vi "Run Sequence.vi"(8 "error in (no error)":errorcluster, 11 "Sequence in":refnum<class "Sequence.lvclass">) -> (0 "error out":errorcluster, 3 "Sequence out":refnum<class "Sequence.lvclass">)   [LabVIEW 2015, in "Mediator.lvlib" / "Sequence.lvclass"]
doc: "This executes the sequence by reserving each step's resources, executing each step, and unreserving each step's resources."
uses:
  Sequence.lvclass
  Sequence.lvclass/Sequence.ctl
  Step/Step.lvclass
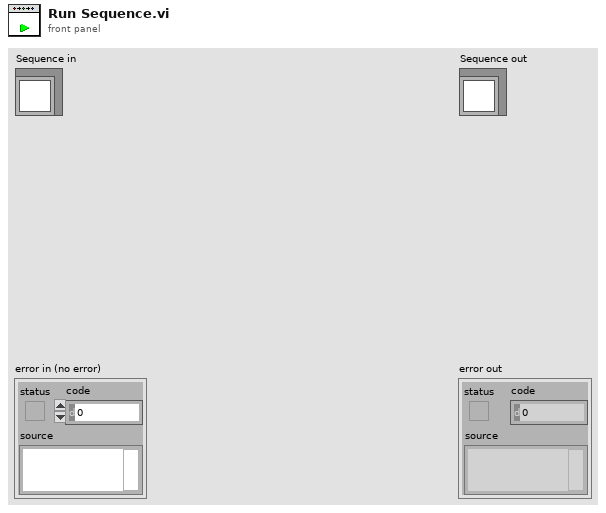
[diagram p1: front panel]
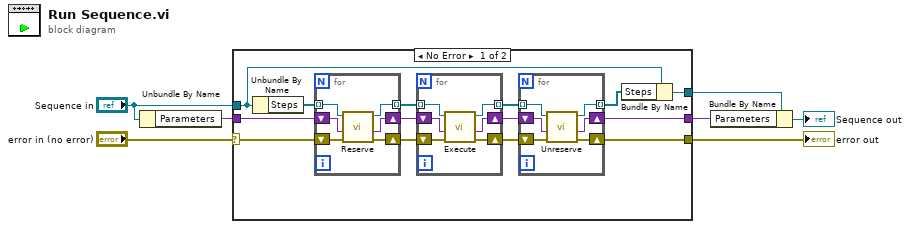
[diagram p0: block diagram]
diagram:
  n1 = Unbundle By Name("Sequence in") -> ("Parameters"=w4:variant)
  n2 = case shown="No Error" "error in (no error)" {
    selector: "error in (no error)" -> [w20 w42]
    tunnel: [w12 w42] -> w6
    tunnel: [w14 w41] -> w3
    tunnel: "Sequence in" -> [w16 w41]
    tunnel: w4 -> [w11 w40]
    tunnel: [w8 w40] -> w1
    frame No Error {
      n3 = Unbundle By Name(w16) -> ("Steps"=w21:refnum<class "Step.lvclass">[])
      n4 = for {
        tunnel: w21 -> [w33] mode=indexing
        shift-right: [w31] -> w19
        shift-left: w20 -> [w32]
        tunnel: [w30] -> w18 mode=indexing
        shift-right: [w28] -> w10
        shift-left: w11 -> [w29]
        n5 = call-dynamic "Reserve.vi"("error in (no error)"=w32, "Sequence Parameters in"=w29, "Step in"=w33) -> ("error out"=w31:errorcluster, "Sequence Parameters out"=w28:variant, "Step out"=w30:refnum<class "Step.lvclass">)  [unwired: 6 in]
      }
      n6 = for {
        tunnel: w18 -> [w39] mode=indexing
        shift-right: [w38] -> w13
        shift-left: w19 -> [w37]
        tunnel: [w36] -> w17 mode=indexing
        shift-right: [w34] -> w9
        shift-left: w10 -> [w35]
        n7 = call-dynamic "Execute.vi"("error in (no error)"=w37, "Sequence Parameters in"=w35, "Step in"=w39) -> ("error out"=w38:errorcluster, "Sequence Parameters out"=w34:variant, "Step out"=w36:refnum<class "Step.lvclass">)  [unwired: 6 in]
      }
      n8 = for {
        tunnel: w17 -> [w27] mode=indexing
        tunnel: [w26] -> w15 mode=indexing
        shift-right: [w24] -> w12
        shift-left: w13 -> [w25]
        shift-right: [w22] -> w8
        shift-left: w9 -> [w23]
        n9 = call-dynamic "Unreserve.vi"("error in (no error)"=w25, "Sequence Parameters in"=w23, "Step in"=w27) -> ("error out"=w24:errorcluster, "Sequence Parameters out"=w22:variant, "Step out"=w26:refnum<class "Step.lvclass">)  [unwired: 6 in]
      }
      n10 = Bundle By Name(cluster=w16, "Steps"=w15) -> (w14:refnum<class "Sequence.lvclass">)
    }
    frame Error {
    }
  }
  "error out" <- w6
  n11 = Bundle By Name(cluster=w3, "Parameters"=w1) -> (→"Sequence out":refnum<class "Sequence.lvclass">)
